vi "Construct - File.vi"(10 "section":string, 11 "config file":path) -> (0 "Error Out":errorcluster, 3 "SQLite Database":refnum<class "SQLite Database.lvclass">)   [LabVIEW 2019, in "TSC Event Logger (SQL).lvlib" / "SQLite Database.lvclass"]
doc: "Construct the database sink type from common ini file format.\n\n<b>Code Developed By:</b>\nTechnology Service Corporation\nBloomington, IN 47403\nwww.tsc.com/atcs\n\nDeveloper:\nDaniel Coons"
uses:
  SQLite Database.lvclass
  C:/Program Files (x86)/National Instruments/LabVIEW 2019/vi.lib/addons/_TSC/TSC Event Logger/Log Sinks/Log Sinks.lvclass
  Layouts/DBLayout/DBLayout.lvclass
  C:/Program Files (x86)/National Instruments/LabVIEW 2019/vi.lib/addons/_TSC/TSC Event Logger/Layouts/Layout.lvclass
  <vilib>/addons/_TSC/TSC Event Logger/Log/Event Level.ctl
  SQLite Database.lvclass/SQLite Database.ctl
  <vilib>/addons/_TSC/TSC Event Logger/Log Sinks/Log Sinks.lvclass/Log Sinks.ctl
  <vilib>/Utility/config.llb/Read Key (Path).vi
  <vilib>/Utility/config.llb/Read Key (String).vi
  <vilib>/Utility/config.llb/Read Key (Double).vi
  <vilib>/Utility/config.llb/Read Key (U32).vi
  <vilib>/Utility/config.llb/Read Key (I32).vi
  <vilib>/Utility/config.llb/NI_LVConfig.lvlib
  <vilib>/addons/_TSC/TSC Event Logger/Log Sinks/Log Sinks.lvclass
  <vilib>/addons/_TSC/TSC Event Logger/TSC Event Logger.lvlib
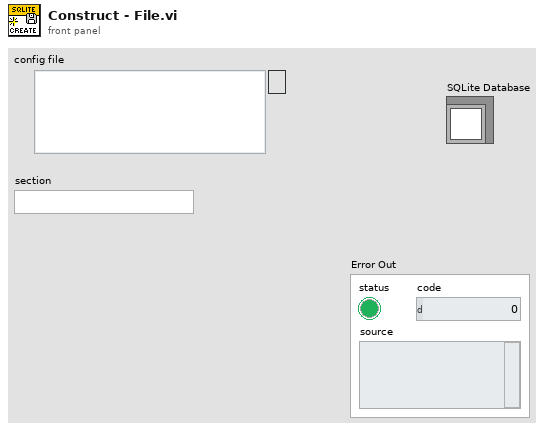
[diagram p1: front panel]
types:
  T1 = typedef "TSC Event Logger.lvlib/Event Level.ctl" = enum16{"OFF", "TRACE", "DEBUG", "INFO", "WARN", "ERROR", "FATAL"}
  T2 = typedef "NI_LVConfig.lvlib/Config Data RefNum.ctl" = refnum<k1>
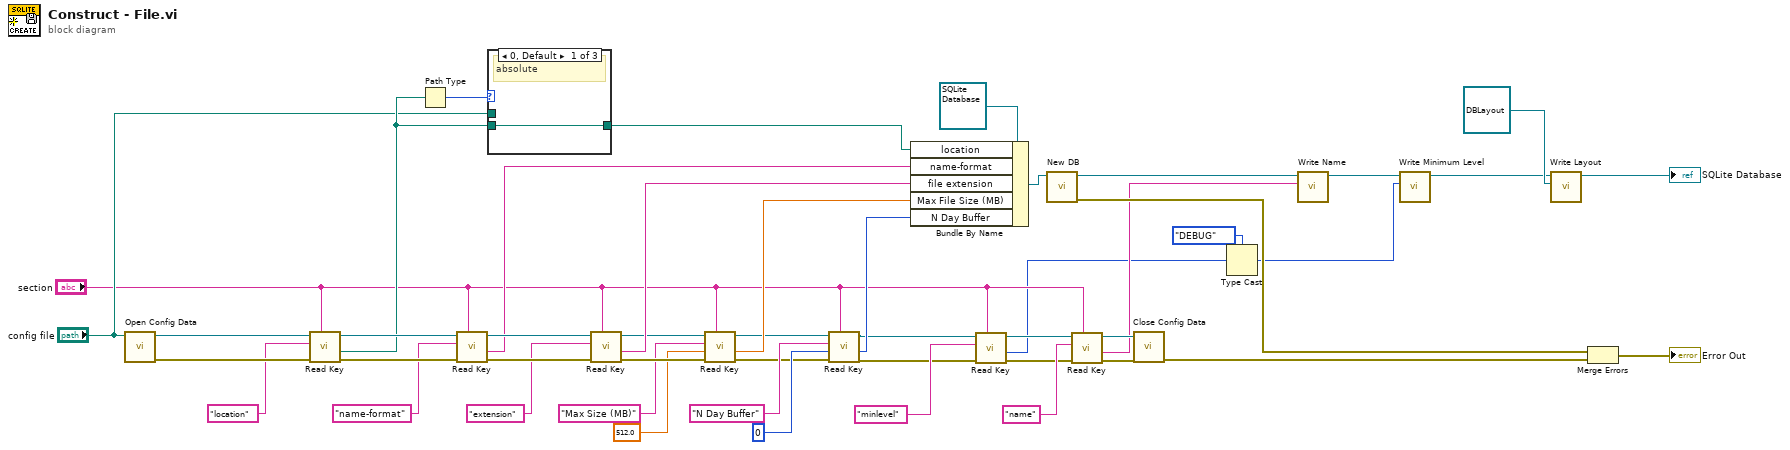
[diagram p0: block diagram]
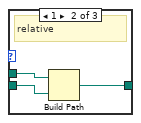
[diagram p2: hidden frame]
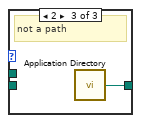
[diagram p3: hidden frame]
diagram:
  n1 = call <vilib>:"Open Config Data.vi"("configuration file path"="config file") -> ("error out"=w47:errorcluster, "refnum"=w45:T2)  [unwired: 8 in, 1 out]
  n2 = call-poly <vilib>:"Read Key.vi"("section"="section", "error in (no error)"=w47, "key"="location", "refnum"=w45) -> ("error out"=w46:errorcluster, "value"=w26:path, "refnum out"=w42:T2)  [unwired: 4 in, 1 out]
  n3 = Path Type(1:w26) -> (0:w27:i16)
  n4 = call-poly <vilib>:"Read Key.vi"("section"="section", "error in (no error)"=w46, "key"="name-format", "refnum"=w42) -> ("error out"=w43:errorcluster, "value"=w34:string, "refnum out"=w39:T2)  [unwired: 4 in, 1 out]
  n5 = case shown="0, Default" w27 {
    tunnel: w26 -> [w49 w51 _]
    tunnel: [w49 w50 w53] -> w25
    tunnel: "config file" -> [_ w52 _]
    frame 0, Default {
      # "absolute"
    }
    frame 1 {
      # "relative"
      n6 = Build Path(base path=w52, name or relative path=w51) -> (appended path=w50:path)
    }
    frame 2 {
      # "not a path"
      n7 = call <vilib>:"Application Directory.vi"() -> ("Application Directory"=w53:path)
    }
  }
  n8 = call-poly <vilib>:"Read Key.vi"("section"="section", "error in (no error)"=w43, "key"="extension", "refnum"=w39) -> ("error out"=w40:errorcluster, "value"=w32:string, "refnum out"=w31:T2)  [unwired: 4 in, 1 out]
  n9 = call-poly <vilib>:"Read Key.vi"("section"="section", "error in (no error)"=w40, "default value"=512.0, "key"="Max Size (MB)", "refnum"=w31) -> ("error out"=w21:errorcluster, "value"=w28:dbl, "refnum out"=w20:T2)  [unwired: 3 in, 1 out]
  n10 = call-poly <vilib>:"Read Key.vi"("section"="section", "error in (no error)"=w21, "default value"=u32 0, "key"="N Day Buffer", "refnum"=w20) -> ("error out"=w10:errorcluster, "value"=w19:u32, "refnum out"=w8:T2)  [unwired: 3 in, 1 out]
  n11 = Bundle By Name(cluster=refnum<class "SQLite Database.lvclass"> refnum ("TSC Event Logger.lvlib:SQLite Database.lvclass"), "location"=w25, "name-format"=w34, "file extension"=w32, "Max File Size (MB)"=w28, "N Day Buffer"=w19) -> (w33:refnum<class "SQLite Database.lvclass">)
  n12 = call-poly <vilib>:"Read Key.vi"("section"="section", "error in (no error)"=w10, "key"="minlevel", "refnum"=w8) -> ("error out"=w11:errorcluster, "value"=w5:i32, "refnum out"=w12:T2)  [unwired: 4 in, 1 out]
  n13 = call "New DB.vi"("SQLite Database in"=w33) -> ("error out"=w36:errorcluster, "SQLite Database out"=w7:refnum<class "SQLite Database.lvclass">)  [unwired: 9 in]
  n14 = call-poly <vilib>:"Read Key.vi"("section"="section", "error in (no error)"=w11, "key"="name", "refnum"=w12) -> ("error out"=w13:errorcluster, "value"=w6:string, "refnum out"=w16:T2)  [unwired: 4 in, 1 out]
  n15 = call <vilib>:"Close Config Data.vi"("error in (no error)"=w13, "refnum"=w16) -> ("error out"=w48:errorcluster)  [unwired: 8 in, 1 out]
  n16 = Type Cast(type=Event_Level."DEBUG" ("Level"), x=w5) -> (*(type *) &x=w2:T1)
  n17 = call <vilib>:"Write Name.vi"("Name"=w6, "Log Sinks in"=w7) -> ("Log Sinks out"=w4:refnum<class "SQLite Database.lvclass">)  [unwired: 9 in]
  n18 = call <vilib>:"Write Minimum Level.vi"("Level"=w2, "Log Sinks in"=w4) -> ("Log Sinks out"=w3:refnum<class "SQLite Database.lvclass">)  [unwired: 9 in]
  n19 = call <vilib>:"Write Layout.vi"("Layout"=refnum<class "DBLayout.lvclass"> refnum ("TSC Event Logger.lvlib:DBLayout.lvclass"), "Log Sinks in"=w3) -> ("Log Sinks out"=→"SQLite Database":refnum<class "SQLite Database.lvclass">)  [unwired: 9 in]
  n20 = Merge Errors(w36, w48) -> (→"Error Out":errorcluster)
